vi "Decode TCP Data - Update.vi"(8 "error in":errorcluster, 9 "Type":string, 10 "Input Data":string) -> (0 "error out":errorcluster, 3 "Data Out":T1)   [LabVIEW 2021]
uses:
  Controls/Host Data Cluster.ctl
  Main Engine/Controls/Main Engine CPU Info.ctl
  Main Engine/Controls/Main Engine CPU JSON.ctl
  Async Serial/Controls/Async Sensor Type.ctl
  <vilib>/measure/madcrms.llb/Averaged DC-RMS for 1 Chan.vi
  <vilib>/addons/_JKI.lib/Serialization/JSON/JKI JSON Serialization.lvlib
  <vilib>/measure/NI_MAPro.lvlib
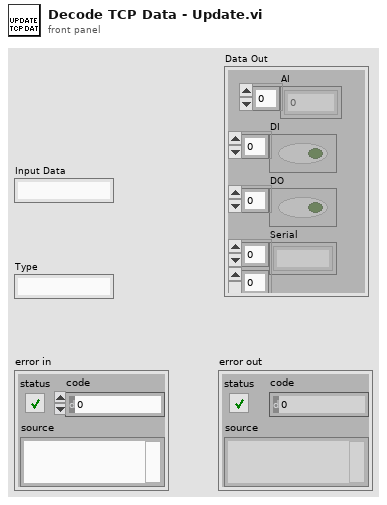
[diagram p1: front panel]
types:
  T1 = typedef "Host Data Cluster.ctl" = cluster{"AI":dbl[], "DI":bool[], "DO":bool[], "Serial":string[][], "CPU":T2, "Stop":bool, "DO Channel":string[]}
  T2 = typedef "Main Engine CPU Info.ctl" = cluster{"Total Load":u32[], "Interrupt Load":u32[], "Total Physical":dbl, "Free Physical":dbl, "Primary Disk Capacity":dbl, "Primary Disk Free":dbl}
  T3 = typedef "Main Engine CPU JSON.ctl" = cluster{"Interface":string, "Interface Data":cluster{"Command":string, "SubCmd":string, "Data":T2, "CPU Frequency":dbl}}
  T4 = cluster{"Command":string, "SubCmd":string, "Channels":string[], "Data":i16[], "Time":string}
  T5 = typedef "Async Sensor Type.ctl" = enum16{"Camera", "INS", "Pri BMS", "Aux BMS", "Depth Sensor", "Altimeter", "OIM", "Thruster", "Acoustic Modem", "LED"}
  T6 = cluster{"Command":string, "SubCmd":string, "Data":cluster{"Channel":string, "Data":waveform(dbl), "Time":timestamp}[]}
  T7 = cluster{"Channel":string, "Data":waveform(dbl), "Time":timestamp}[]
  T8 = cluster{"Command":string, "SubCmd":string, "Data":cluster{"Port":string, "Length":u16, "Data":u8[], "Time":string}}
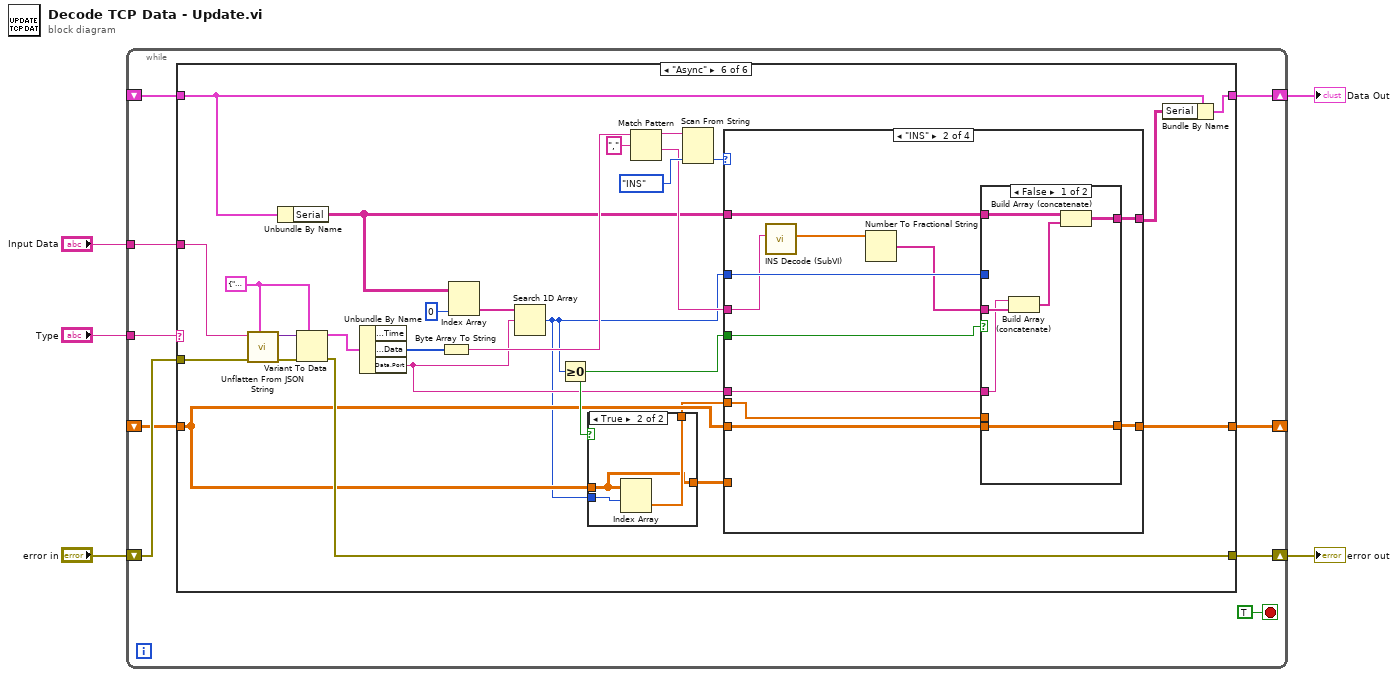
[diagram p0: block diagram]
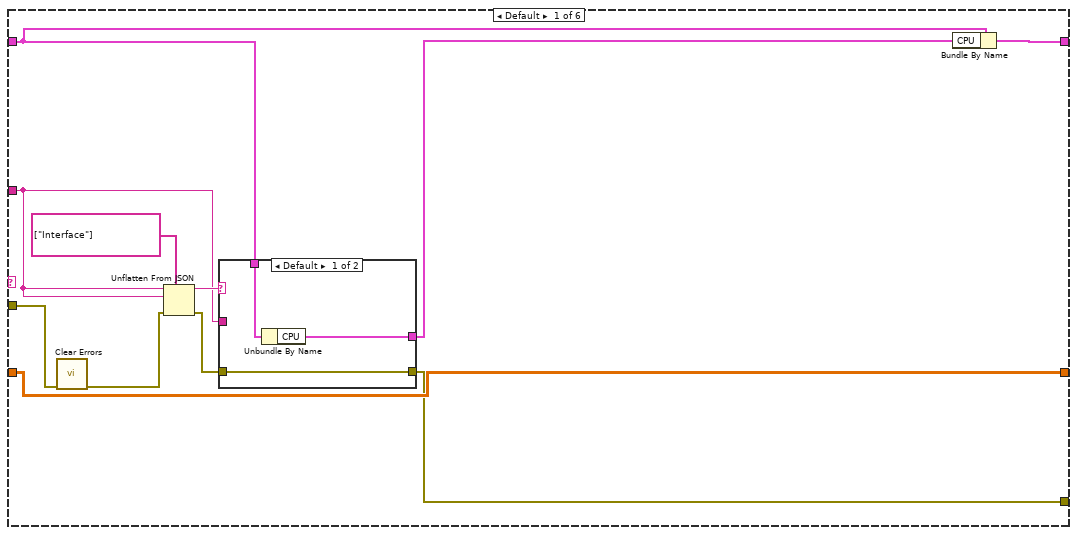
[diagram p2: hidden frame]
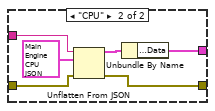
[diagram p3: hidden frame]
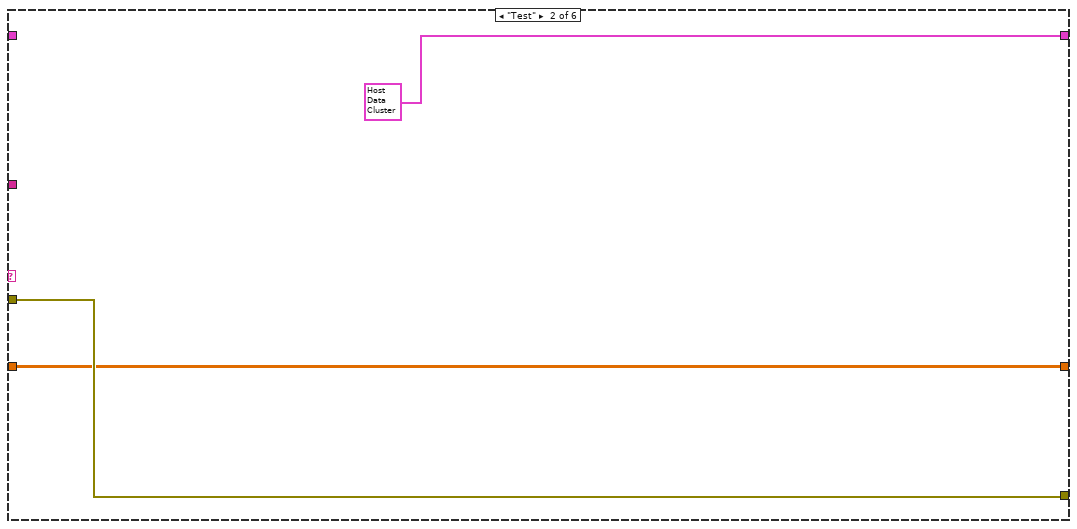
[diagram p4: hidden frame]
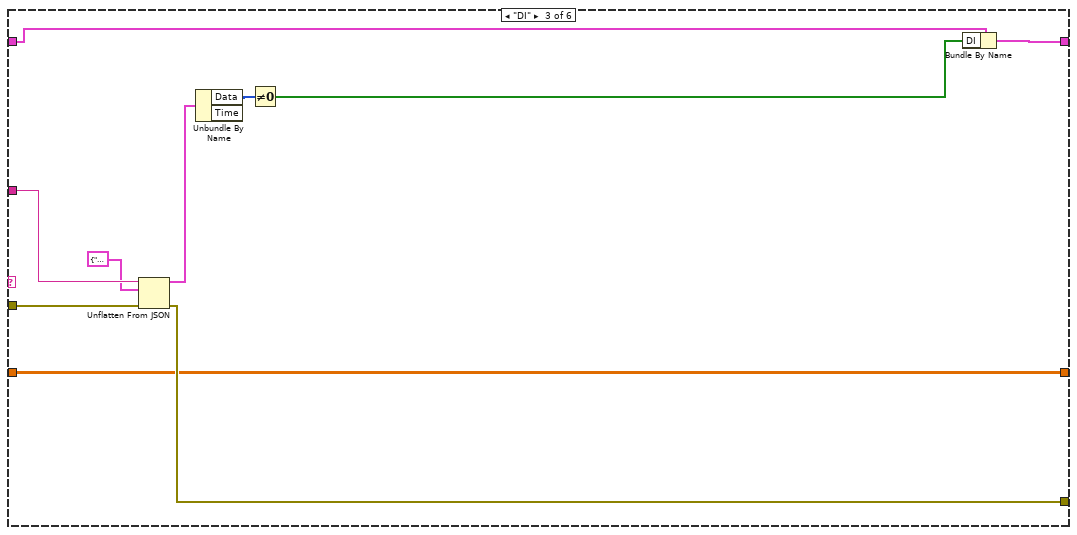
[diagram p5: hidden frame]
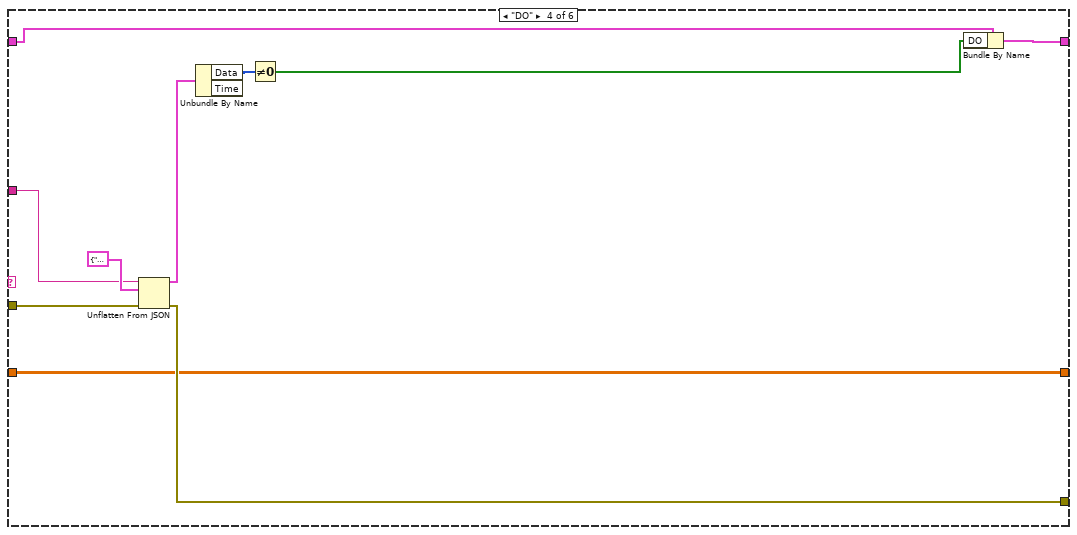
[diagram p6: hidden frame]
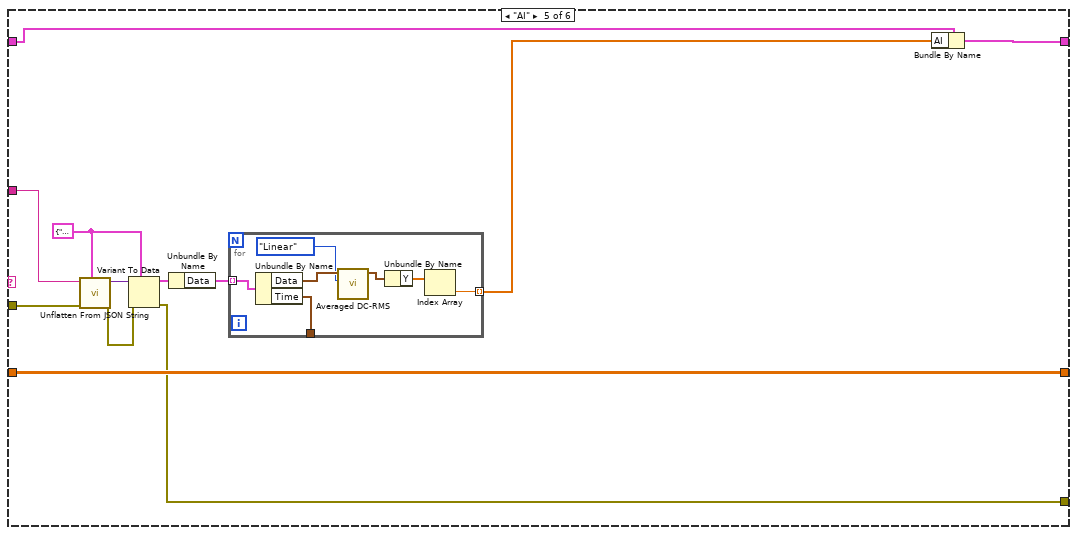
[diagram p7: hidden frame]
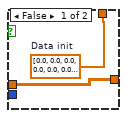
[diagram p8: hidden frame]
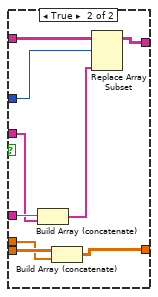
[diagram p10: hidden frame]
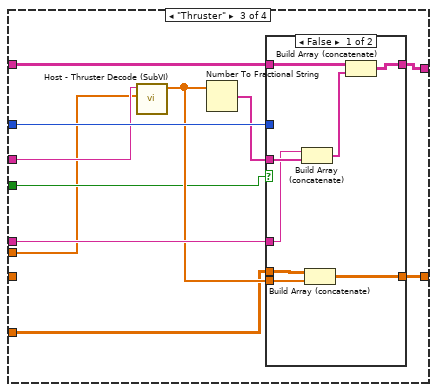
[diagram p11: hidden frame]
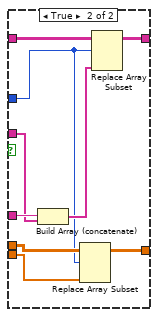
[diagram p12: hidden frame]
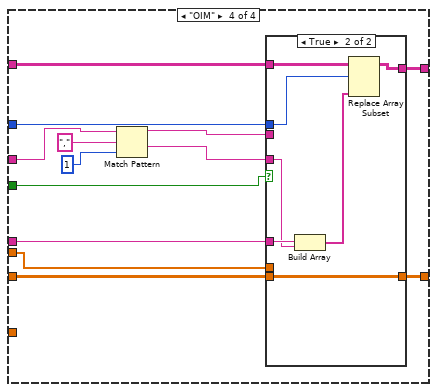
[diagram p13: hidden frame]
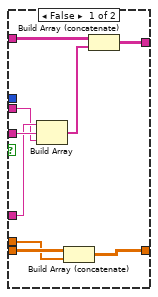
[diagram p14: hidden frame]
diagram:
  n1 = while {
    tunnel: "Input Data" -> [w14]
    tunnel: "Type" -> [w12]
    shift-right: [w6] -> w5
    shift-left: "error in" -> [w13]
    shift-right: [w10] -> w1
    shift-left: _ -> [w11]
    shift-right: [w8] -> _
    shift-left: _ -> [w7]
    stop <- TRUE stop-if-true
    n2 = case shown="\"Async\"" w12 {
      tunnel: w14 -> [w22 _ w47 w49 w69 w103]
      tunnel: w13 -> [w23 w37 w46 w57 w68 w102]
      tunnel: [w15 w37 w42 w54 w58 w98] -> w6
      tunnel: w11 -> [w18 _ w41 w51 w62 w93]
      tunnel: [w19 T1 {"AI"=[], "DI"=[], "DO"=[], "Serial"=[], "CPU"={"Total Load"=[], "Interrupt Load"=[], "Total Physical"=0.0, "Free Physical"=0.0, "Primary Disk Capacity"=0.0, "Primary Disk Free"=0.0}, "Stop"=FALSE, "DO Channel"=[]} ("Data Out") w39 w50 w60 w95] -> w10
      tunnel: [w16 w35 w38 w48 w59 w81] -> w8
      tunnel: w7 -> [w16 w35 w38 w48 w59 w80]
      frame Default {
        n3 = call <vilib>:"Clear Errors.vi"("error in (no error)"=w23) -> ("error out"=w21:errorcluster)  [unwired: 5 in, 1 out]
        n4 = Unflatten From JSON(path=string[] ["Interface"], JSON string=w22, type and defaults=w22, error in (no error)=w21) -> (value=w24:string, error out=w20:errorcluster)  [unwired: 3 in]
        n5 = case shown="Default" w24 {
          tunnel: w22 -> [_ w34]
          tunnel: w20 -> [w28 w33]
          tunnel: [w28 w32] -> w15
          tunnel: [w26 w29] -> w17
          tunnel: w18 -> [w27 _]
          frame Default {
            n6 = Unbundle By Name(w27) -> ("CPU"=w26:T2)
          }
          frame "CPU" {
            n7 = Unflatten From JSON(JSON string=w34, type and defaults=T3 {"Interface"="CPU", "Interface Data"={"Command"="CPU Info", "SubCmd"="Monitor", "Data"={"Total Load"=[], "Interrupt Load"=[], "Total Physical"=0.0, "Free Physical"=0.0, "Primary Disk Capacity"=0.0, "Primary Disk Free"=0.0}, "CPU Frequency"=0.0}}, error in (no error)=w33) -> (value=w31:T3, error out=w32:errorcluster)  [unwired: 4 in]
            n8 = Unbundle By Name(w31) -> ("Interface Data.Data"=w29:T2)
          }
        }
        n9 = Bundle By Name(cluster=w18, "CPU"=w17) -> (w19:T1)
      }
      frame "Test" {
      }
      frame "DI" {
        n10 = Unflatten From JSON(JSON string=w47, type and defaults=T4 {"Command"="", "SubCmd"="", "Channels"=[], "Data"=[], "Time"=""} ("cluster"), error in (no error)=w46) -> (value=w44:T4, error out=w42:errorcluster)  [unwired: 4 in]
        n11 = Unbundle By Name(w44) -> ("Data"=w43:i16[])  [unwired: 1 out]
        n12 = Not Equal To 0?(x=w43) -> (x != 0?=w40:bool[])
        n13 = Bundle By Name(cluster=w41, "DI"=w40) -> (w39:T1)
      }
      frame "DO" {
        n14 = Unflatten From JSON(JSON string=w49, type and defaults=T4 {"Command"="", "SubCmd"="", "Channels"=[], "Data"=[], "Time"=""} ("cluster"), error in (no error)=w57) -> (value=w52:T4, error out=w54:errorcluster)  [unwired: 4 in]
        n15 = Unbundle By Name(w52) -> ("Data"=w55:i16[])  [unwired: 1 out]
        n16 = Not Equal To 0?(x=w55) -> (x != 0?=w53:bool[])
        n17 = Bundle By Name(cluster=w51, "DO"=w53) -> (w50:T1)
      }
      frame "AI" {
        w64 = T6 {"Command"="AI", "SubCmd"="Monitoring", "Data"=[]} ("cluster")
        n18 = call <vilib>:"Unflatten From JSON String.vi"("Type and Defaults"=w64, "error in"=w68, "JSON String"=w69) -> ("error out"=w67:errorcluster, "Variant"=w66:variant)  [unwired: 7 in]
        n19 = Variant To Data(error in=w67, type=w64, Variant=w66) -> (data=w65:T6, error out=w58:errorcluster)
        n20 = Unbundle By Name(w65) -> ("Data"=w63:T7)
        n21 = for {
          tunnel: w63 -> [w76] mode=indexing
          tunnel: [w75] -> w61 mode=indexing
          tunnel: [w73] -> _
          n22 = Unbundle By Name(w76) -> ("Data"=w72:waveform(dbl), "Time"=w73:timestamp)
          n23 = call-poly <vilib>:"Averaged DC-RMS.vi"("averaging type"=enum16{"Linear", "Exponential"}."Linear", "signal in"=w72) -> ("DC value waveform"=w70:waveform(dbl))  [unwired: 5 in, 4 out]
          n24 = Unbundle By Name(w70) -> ("Y"=w74:dbl[])
          n25 = Index Array(array=w74) -> (element=w75:dbl)  [unwired: 1 in]
        }
        n26 = Bundle By Name(cluster=w62, "AI"=w61) -> (w60:T1)
      }
      frame "Async" {
        w97 = T8 {"Command"="", "SubCmd"="", "Data"={"Port"="", "Length"=0, "Data"=[], "Time"=""}}
        n27 = call <vilib>:"Unflatten From JSON String.vi"("Type and Defaults"=w97, "error in"=w102, "JSON String"=w103) -> ("error out"=w101:errorcluster, "Variant"=w100:variant)  [unwired: 7 in]
        n28 = Unbundle By Name(w93) -> ("Serial"=w86:string[][])
        n29 = Variant To Data(error in=w101, type=w97, Variant=w100) -> (data=w84:T8, error out=w98:errorcluster)
        n30 = Unbundle By Name(w84) -> ("Data.Data"=w99:u8[], "Data.Port"=w85:string)  [unwired: 1 out]
        n31 = Byte Array To String(unsigned byte array=w99) -> (string=w89:string)
        n32 = Index Array(array=w86, index (col)=0 ("disabled index (col)")) -> (element=w82:string[])  [unwired: 1 in]
        n33 = Search 1D Array(1D array=w82, element=w85) -> (index of element=w79:i32)  [unwired: 1 in]
        n34 = Greater Or Equal To 0?(x=w79) -> (x >= 0?=w96:bool)
        n35 = case shown="True" w96 {
          tunnel: [w105 w107] -> w77
          tunnel: w80 -> [w104 w106]
          tunnel: w79 -> [_ w108]
          tunnel: [w104 w106] -> w78
          frame False {
            w105 = dbl[] [0.0, 0.0, 0.0, 0.0, 0.0, 0.0, 0.0, 0.0, 0.0, 0.0, 0.0]  # Data init
          }
          frame True {
            n36 = Index Array(array=w106, index (row)=w108) -> (element=w107:dbl[])  [unwired: 1 in]
          }
        }
        n37 = Match Pattern(string=w89, regular expression=",") -> (before substring=w92:string, after substring=w87:string)  [unwired: 1 in, 2 out]
        n38 = Scan From String(input string=w92, default 1=Async_Sensor_Type."INS" ("Sensor Type")) -> (output 1=w88:T5)  [unwired: 3 in, 3 out]
        n39 = case shown="\"INS\"" w88 {
          tunnel: w96 -> [_ w121 w139 w177]
          tunnel: w79 -> [_ w120 w147 w176]
          tunnel: w85 -> [_ w119 w146 w175]
          tunnel: [w110 w118 w145 w174] -> w94
          tunnel: w86 -> [w110 w117 w144 w173]
          tunnel: w87 -> [_ w116 w142 w170]
          tunnel: [w109 w112 w140 w166] -> w81
          tunnel: w80 -> [w109 w113 _ w167]
          tunnel: w77 -> [_ w111 w138 w165]
          tunnel: w78 -> [_ _ w137 _]
          frame Default {
          }
          frame "INS" {
            n40 = call "INS Decode (SubVI).vi"("read buffer"=w116) -> ("Data out"=w115:dbl[])  [unwired: 10 in]
            n41 = Number To Fractional String(number=w115) -> (F-format string=w114:string[])  [unwired: 3 in]
            n42 = case shown="False" w121 {
              tunnel: w114 -> [w126 w133]
              tunnel: w117 -> [w127 w136]
              tunnel: w120 -> [_ w135]
              tunnel: w119 -> [w125 w134]
              tunnel: [w124 w132] -> w118
              tunnel: w113 -> [w122 w130]
              tunnel: [w122 w129] -> w112
              tunnel: w111 -> [_ w128]
              frame False {
                n43 = Build Array (concatenate)(w125, w126) -> (w123:string[])
                n44 = Build Array (concatenate)(w127, w123) -> (w124:string[][])
              }
              frame True {
                n45 = Build Array (concatenate)(w134, w133) -> (w131:string[])
                n46 = Build Array (concatenate)(w130, w128) -> (w129:dbl[][])
                n47 = Replace Array Subset(array=w136, new element=w131, index (row)=w135) -> (w132:string[][])  [unwired: 1 in]
              }
            }
          }
          frame "Thruster" {
            n48 = call "Host - Thruster Decode (SubVI).vi"("Array"=w138, "read buffer"=w142) -> ("Data init out"=w141:dbl[])  [unwired: 9 in]
            n49 = Number To Fractional String(number=w141) -> (F-format string=w143:string[])  [unwired: 3 in]
            n50 = case shown="False" w139 {
              tunnel: w143 -> [w154 w162]
              tunnel: w144 -> [w155 w164]
              tunnel: w147 -> [_ w157]
              tunnel: w146 -> [w153 w163]
              tunnel: [w152 w161] -> w145
              tunnel: w141 -> [w150 w156]
              tunnel: [w149 w158] -> w140
              tunnel: w137 -> [w148 w159]
              frame False {
                n51 = Build Array (concatenate)(w153, w154) -> (w151:string[])
                n52 = Build Array (concatenate)(w148, w150) -> (w149:dbl[][])
                n53 = Build Array (concatenate)(w155, w151) -> (w152:string[][])
              }
              frame True {
                n54 = Build Array (concatenate)(w163, w162) -> (w160:string[])
                n55 = Replace Array Subset(array=w159, new element=w156, index (row)=w157) -> (w158:dbl[][])  [unwired: 1 in]
                n56 = Replace Array Subset(array=w164, new element=w160, index (row)=w157) -> (w161:string[][])  [unwired: 1 in]
              }
            }
          }
          frame "OIM" {
            n57 = Match Pattern(string=w170, regular expression=",", offset (0)=1) -> (before substring=w168:string, after substring=w169:string)  [unwired: 2 out]
            n58 = case shown="True" w177 {
              tunnel: w169 -> [w185 w190]
              tunnel: w173 -> [w186 w193]
              tunnel: w176 -> [_ w192]
              tunnel: w175 -> [w184 w191]
              tunnel: [w183 w189] -> w174
              tunnel: w168 -> [w181 _]
              tunnel: w167 -> [w180 w187]
              tunnel: [w179 w187] -> w166
              tunnel: w165 -> [w178 _]
              frame False {
                n59 = Build Array(w184, w185, w181) -> (w182:string[])
                n60 = Build Array (concatenate)(w180, w178) -> (w179:dbl[][])
                n61 = Build Array (concatenate)(w186, w182) -> (w183:string[][])
              }
              frame True {
                n62 = Build Array(w191, w190) -> (w188:string[])
                n63 = Replace Array Subset(array=w193, new element=w188, index (row)=w192) -> (w189:string[][])  [unwired: 1 in]
              }
            }
          }
        }
        n64 = Bundle By Name(cluster=w93, "Serial"=w94) -> (w95:T1)
      }
    }
  }
  "error out" <- w5
  "Data Out" <- w1
